vi "Execute.vi"(8 "error in (no error)":errorcluster, 11 "CIFTemplatePlugin in":refnum<class "CIFTemplatePlugin.lvclass">) -> (0 "error out":errorcluster, 3 "CIFTemplatePlugin out":refnum<class "CIFTemplatePlugin.lvclass">)   [LabVIEW 2021, in "CIFTemplatePlugin.lvclass"]
uses:
  CIFTemplatePlugin.lvclass
  D:/dev/CIF-LVCore/src/CIFCore/Class/CIFCorePlugin.lvclass
  CIFCore/Class/CIFCorePlugin.lvclass/CIFCorePlugin.ctl
  CIFCore/Class/Typedef/Energized States.ctl
  CIFTemplatePlugin.lvclass/CIFTemplatePlugin.ctl
  Channels/CIFChannelMng/CIFChannelMng.lvclass/CIFChannelMng.ctl
  CIFUtilities/CIFClocks/Core/Get Time.vi
  CIFCore/Class/Accessors/Timestamps/Write Execute TS.vi
  CIFUtilities/CIFClocks/Core/Sleep Until Future Time.vi
  <vilib>/Utility/error.llb/Clear Errors.vi
  CIFCore/Class/Accessors/Read Sleep Limits (ns).vi
  CIFCore/Class/Accessors/Timestamps/Write Target Wake TS.vi
  CIFCore/Class/SubVIs/Start Running.vi
  CIFCore/Common/Utilities/Add Error.vi
  CIFCore/Class/Accessors/Read Plugin Name.vi
  CIFCore/Class/Accessors/Get Time.vi
  CIFCore/Class/Accessors/Timestamps/Read Running TS.vi
  CIFCore/Class/Accessors/Read Running Internal Data.vi
  CIFCore/Class/Accessors/Read Timing Override.vi
  CIFCore/Class/Accessors/Read Common Config.vi
  CIFCore/Class/Channel RW/Read Double.vi
  CIFCore/Class/Channel RW/Write Double.vi
  CIFCore/Class/Channel RW/Read U64.vi
  CIFCore/Class/Channel RW/Write U64.vi
  CIFCore/Class/Accessors/Monitor/Write Double 1.vi
  CIFCore/Class/Accessors/Monitor/Write U64 1.vi
  CIFCore/Class/Accessors/Monitor/Write I64 1.vi
  CIFCore/Class/Accessors/Monitor/Write I64 2.vi
  CIFUtilities/CIFClocks/Time Conversion/LabVIEW Time to UTC Time.vi
  CIFCore/Common/Utilities/Append Error Location.vi
  Channels/CIFChannelMng/Accessors/Read Channel Array.vi
  Channels/CIFChannelMng/Accessors/Write Channel Array.vi
  Channels/CIFChannels/CIFChannels.lvclass
  CIFCore/Class/CIFCorePlugin.lvclass
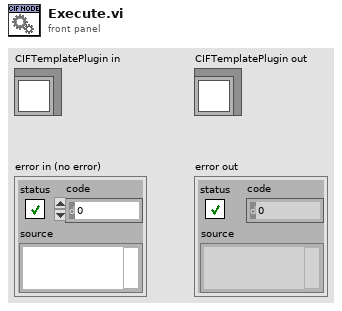
[diagram p1: front panel]
types:
  T1 = typedef "CIFCorePlugin.lvclass/Energized States.ctl" = enum16{"Listen", "Prepare", "Execute", "Housekeep", "Cleanup", "Destroy"}
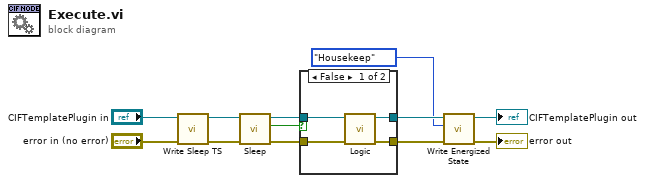
[diagram p0: block diagram]
diagram:
  n1 = call "Write Sleep TS.vi"("error in (no error)"="error in (no error)", "CIFCorePlugin in"="CIFTemplatePlugin in") -> ("error out"=w8:errorcluster, "CIFCorePlugin out"=w9:refnum<class "CIFTemplatePlugin.lvclass">)  [unwired: 8 in]
  n2 = call "Sleep.vi"("error in (no error)"=w8, "CIFCorePlugin in"=w9) -> ("error out"=w10:errorcluster, "Housekeep only"=w7:bool, "CIFCorePlugin out"=w11:refnum<class "CIFTemplatePlugin.lvclass">)  [unwired: 7 in]
  n3 = case shown="False" w7 {
    tunnel: [w13 w17] -> w2
    tunnel: [w14 w18] -> w5
    tunnel: w11 -> [w15 w18]
    tunnel: w10 -> [w16 w17]
    frame False {
      n4 = call "Logic.vi"("error in (no error)"=w16, "CIFTemplatePlugin in"=w15) -> ("error out"=w13:errorcluster, "CIFTemplatePlugin out"=w14:refnum<class "CIFTemplatePlugin.lvclass">)  [unwired: 8 in]
    }
    frame True {
    }
  }
  n5 = call "Write Energized State.vi"("error in (no error)"=w2, "Energized State"=Energized_States."Housekeep", "CIFCorePlugin in"=w5) -> ("error out"=→"error out":errorcluster, "CIFCorePlugin out"=→"CIFTemplatePlugin out":refnum<class "CIFTemplatePlugin.lvclass">)  [unwired: 7 in]
